vi "add-titel.vi"(0 "deutsch?":bool, 1 "abposeinfügen":bool, 2 "input-array":string[](array[string]), 5 "pfade":string[](array[string]), 7 "use input-array?":bool, 9 "playlist":string[](array[string]), 11 "symbole":dbl[](array[numeric]), 12 "pos":dbl, 13 "dateitypen":string) -> (4 "pfade out":string[](array[string]), 6 "playlist out":string[](array[string]), 10 "symbole out":dbl[](array[numeric]))   [LabVIEW 2012]
uses:
  <vilib>/Utility/error.llb/DialogType.ctl
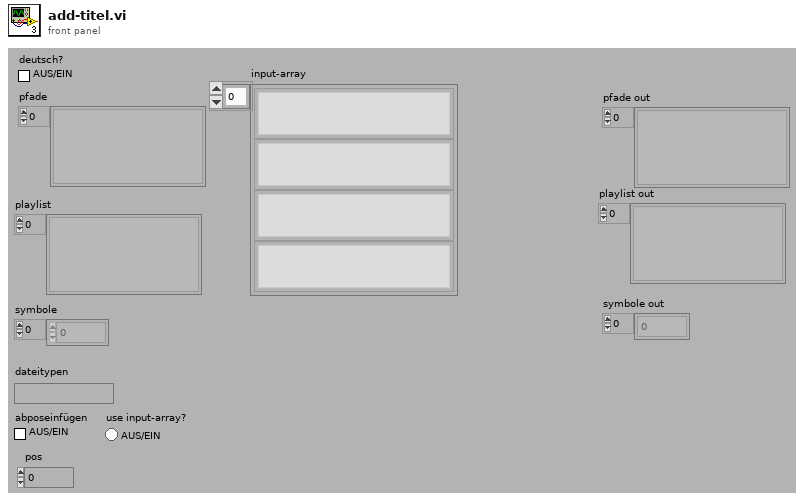
[diagram p1: front panel]
types:
  T1 = typedef "DialogType.ctl" = u16
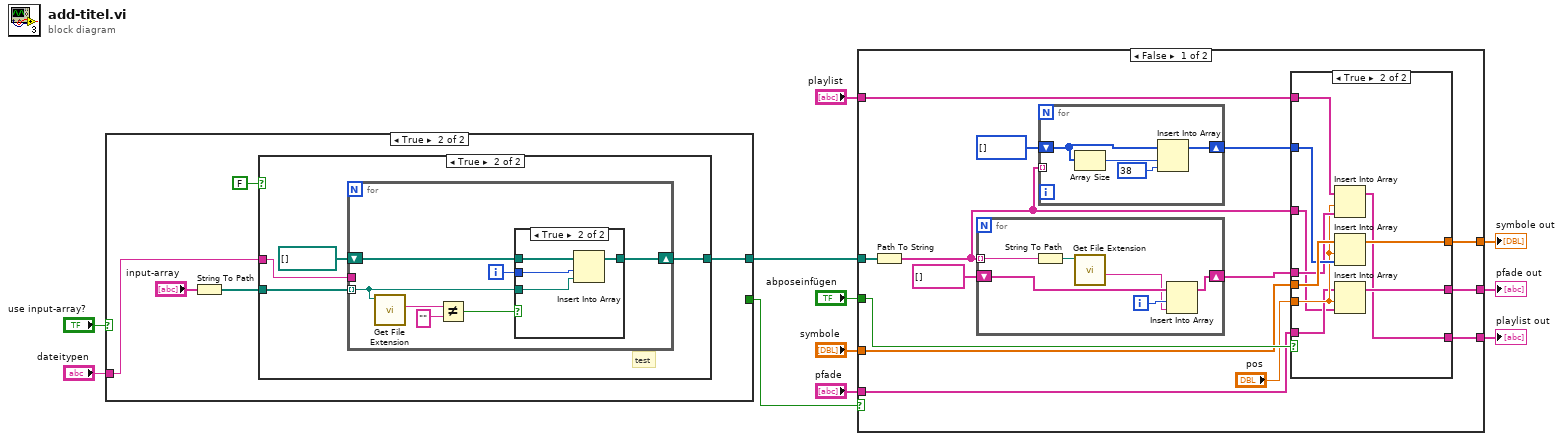
[diagram p0: block diagram]
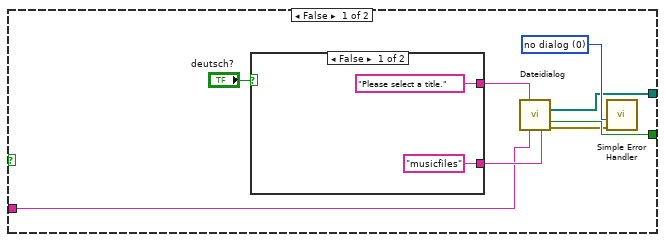
[diagram p2: hidden frame]
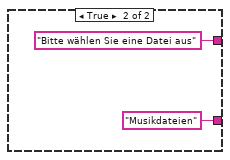
[diagram p3: hidden frame]
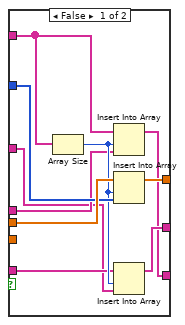
[diagram p6: hidden frame]
diagram:
  n1 = case shown="True" "use input-array?" {
    tunnel: [w16 _] -> w11
    tunnel: [w13 w25] -> w10
    tunnel: "dateitypen" -> [w12 w26]
    frame False {
      w14 = T1 0 items=["no dialog", "OK message", "continue or stop message", "OK message + warnings", "continue/stop + warnings"] ("type of dialog (OK msg:1)")
      n2 = case shown="False" "deutsch?" {
        tunnel: ["Please select a title." ("Eingabeaufforderung") "Bitte wählen Sie eine Datei aus" ("Eingabeaufforderung")] -> w18
        tunnel: ["musicfiles" "Musikdateien"] -> w19
        frame False {
        }
        frame True {
        }
      }
      n3 = call "Dateidialog"("prompt"=w18, "pattern (all files)"=w12, "pattern label"=w19) -> ("selected paths"=w13:path[], "cancelled"=w16:bool, "error out"=w15:errorcluster)  [unwired: 4 in, 6 out]
      n4 = call <vilib>:"Simple Error Handler.vi"("type of dialog (OK msg:1)"=w14, "error in (no error)"=w15) -> ()  [unwired: 1 in, 7 out]
    }
    frame True {
      n5 = String To Path(string="input-array") -> (path=w27:path[])
      n6 = case shown="True" FALSE {
        tunnel: w27 -> [w29 w33]
        tunnel: w26 -> [_ w31]
        tunnel: [w29 w30] -> w25
        frame False {
        }
        frame True {
          # "test"
          n7 = for {
            tunnel: w33 -> [w36] mode=indexing
            shift-right: [w37] -> w30
            shift-left: path[] [] -> [w40]
            tunnel: w31 -> [_]
            i -> [w39]
            n8 = call <vilib>:"Get File Extension.vi"("file"=w36) -> ("lowercase file extension"=w34:string)  [unwired: 7 in, 3 out]
            n9 = Not Equal?(x=w34, y="" ("lowercase file extension")) -> (x != y?=w38:bool)
            n10 = case shown="True" w38 {
              tunnel: w40 -> [w41 w45]
              tunnel: w39 -> [_ w44]
              tunnel: [w41 w43] -> w37
              tunnel: w36 -> [_ w42]
              frame False {
              }
              frame True {
                n11 = Insert Into Array(array=w45, index=w44, new element=w42) -> (w43:path[])
              }
            }
          }
        }
      }
    }
  }
  n12 = case shown="False" w11 {
    tunnel: w10 -> [w58 _]
    tunnel: [w47 w90] -> w3
    tunnel: "abposeinfügen" -> [w57 _]
    tunnel: [w55 w92] -> w8
    tunnel: "symbole" -> [w54 w92]
    tunnel: "playlist" -> [w51 w91]
    tunnel: [w50 w91] -> w5
    tunnel: "pfade" -> [w49 w90]
    frame False {
      n13 = Path To String(path=w58) -> (string=w48:string[])
      n14 = for {
        tunnel: w48 -> [w65] mode=indexing
        shift-right: [w60] -> w52
        shift-left: string[] [] -> [w63]
        i -> [w62]
        n15 = String To Path(string=w65) -> (path=w64:path)
        n16 = call <vilib>:"Get File Extension.vi"("file"=w64) -> ("filename without extension"=w61:string)  [unwired: 7 in, 3 out]
        n17 = Insert Into Array(array=w63, index=w62, new element=w61) -> (w60:string[])
      }
      n18 = for {
        shift-right: [w87] -> w56
        shift-left: i32[] [] -> [w88]
        tunnel: w48 -> [_] mode=indexing
        n19 = Array Size(array=w88) -> (size(s)=w89:i32)
        n20 = Insert Into Array(array=w88, index=w89, new element=38) -> (w87:i32[])
      }
      n21 = case shown="True" w57 {
        tunnel: w48 -> [w66 w76]
        tunnel: w49 -> [w67 w77]
        tunnel: [w75 w85] -> w47
        tunnel: w54 -> [w74 w84]
        tunnel: w56 -> [w73 w83]
        tunnel: [w72 w82] -> w55
        tunnel: w51 -> [w68 w81]
        tunnel: [w69 w80] -> w50
        tunnel: w52 -> [w70 w79]
        tunnel: "pos" -> [_ w78]
        frame False {
          n22 = Array Size(array=w68) -> (size(s)=w71:i32)
          n23 = Insert Into Array(array=w68, index=w71, new element=w70) -> (w69:string[])
          n24 = Insert Into Array(array=w74, index=w71, new element=w73) -> (w72:dbl[])
          n25 = Insert Into Array(array=w67, index=w71, new element=w66) -> (w75:string[])
        }
        frame True {
          n26 = Insert Into Array(array=w81, index=w78, new element=w79) -> (w80:string[])
          n27 = Insert Into Array(array=w84, index=w78, new element=w83) -> (w82:dbl[])
          n28 = Insert Into Array(array=w77, index=w78, new element=w76) -> (w85:string[])
        }
      }
    }
    frame True {
    }
  }
  "pfade out" <- w3
  "playlist out" <- w5
  "symbole out" <- w8
